vi "Sequence.vi"() -> ()   [LabVIEW 2019]
panel:
  in  "Array":dbl[](array[numeric])
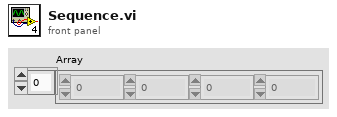
[diagram p1: front panel]
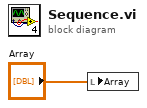
[diagram p0: block diagram]
diagram:
  n1 = local write "Array"("Array") -> ()
